vi "Tool Object.vi"(8 "error in (no error)":errorcluster, 11 "Tool Path in":refnum<class "Tool Path.lvclass">) -> (0 "error out":errorcluster, 2 "Points":T1[](array[typedef]), 3 "Tool Path out":refnum<class "Tool Path.lvclass">)   [LabVIEW 2019, in "Tool Path.lvclass"]
uses:
  Tool Path.lvclass
  Parse/PathCommands/Point.ctl
  Settings/ObjectSettings/ObjectSettings.lvclass/ObjectSettings.ctl
  Settings/Path Settings/Path Settings.lvclass
  C:/Users/Albro/Documents/GitHub/AFM-Lithography/lvsrc/Classes/Settings/ObjectSettings/ObjectSettings.lvclass
  Settings/ObjectSettings/ObjectSettings.lvclass
  Parse/PathCommands/PathCommands.lvclass
panel:
  out "Voltage Values":dbl[](array[numeric])
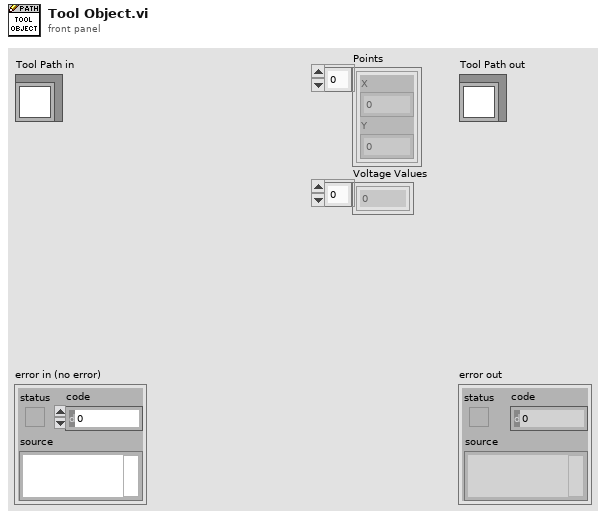
[diagram p1: front panel]
types:
  T1 = typedef "PathCommands.lvclass/Point.ctl" = cluster{"X":dbl, "Y":dbl}
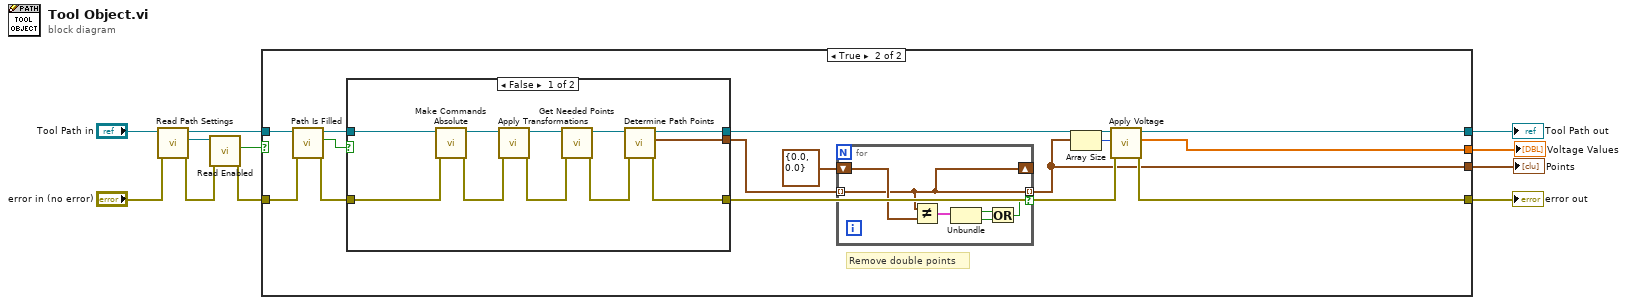
[diagram p0: block diagram]
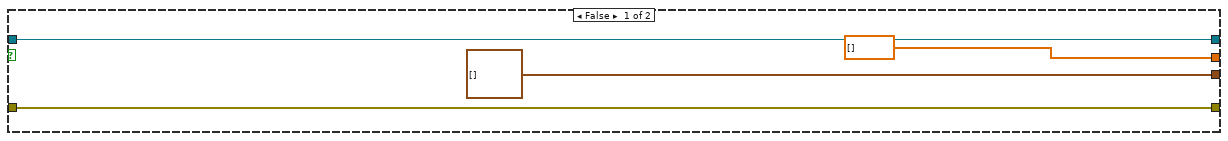
[diagram p2: hidden frame]
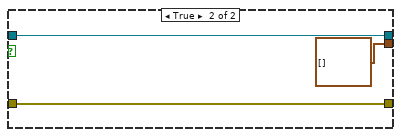
[diagram p3: hidden frame]
diagram:
  n1 = call-dynamic "Read Path Settings.vi"("error in (no error)"="error in (no error)", "Tool Path in"="Tool Path in") -> ("error out"=w4:errorcluster, "Path Settings.lvclass"=w10:refnum<class "Path Settings.lvclass">, "Tool Path out"=w9:refnum<class "Tool Path.lvclass">)  [unwired: 7 in]
  n2 = call "Read Enabled.vi"("error in (no error)"=w4, "ObjectSettings in"=w10) -> ("error out"=w3:errorcluster, "Enabled"=w6:bool)  [unwired: 7 in, 1 out]
  n3 = case shown="True" w6 {
    tunnel: w9 -> [w15 w28]
    tunnel: [w15 w23] -> w8
    tunnel: w3 -> [w14 w25]
    tunnel: [w14 w21] -> w7
    tunnel: [T1[] [] ("Points") w18] -> w2
    tunnel: [dbl[] [] ("Voltage Values") w16] -> w1
    frame False {
    }
    frame True {
      # "Remove double points"
      n4 = call "Path Is Filled.vi"("error in (no error)"=w25, "Tool Path in"=w28) -> ("error out"=w26:errorcluster, "Filled?"=w27:bool, "Tool Path out"=w29:refnum<class "Tool Path.lvclass">)  [unwired: 7 in]
      n5 = case shown="False" w27 {
        tunnel: w29 -> [w46 w49]
        tunnel: [w42 w49] -> w24
        tunnel: w26 -> [w41 w48]
        tunnel: [w37 w48] -> w22
        tunnel: [w36 T1[] [] ("Points")] -> w17
        frame False {
          n6 = call "Make Commands Absolute.vi"("error in (no error)"=w41, "Tool Path in"=w46) -> ("error out"=w40:errorcluster, "Tool Path out"=w43:refnum<class "Tool Path.lvclass">)  [unwired: 8 in]
          n7 = call-dynamic "Apply Transformations.vi"("error in (no error)"=w40, "Tool Path in"=w43) -> ("error out"=w39:errorcluster, "Tool Path out"=w45:refnum<class "Tool Path.lvclass">)  [unwired: 8 in]
          n8 = call-dynamic "Get Needed Points.vi"("error in (no error)"=w39, "Tool Path in"=w45) -> ("error out"=w38:errorcluster, "Tool Path out"=w44:refnum<class "Tool Path.lvclass">)  [unwired: 8 in]
          n9 = call-dynamic "Determine Path Points.vi"("error in (no error)"=w38, "Tool Path in"=w44) -> ("error out"=w37:errorcluster, "Points"=w36:T1[], "Tool Path out"=w42:refnum<class "Tool Path.lvclass">)  [unwired: 7 in]
        }
        frame True {
        }
      }
      n10 = for {
        tunnel: w17 -> [w34] mode=indexing
        tunnel: [w34] -> w18 mode=indexing if=w30
        shift-right: [w34] -> _
        shift-left: T1 {"X"=0.0, "Y"=0.0} ("Point") -> [w35]
        n11 = Not Equal?(x=w34, y=w35) -> (x != y?=w33:cluster{"X":bool, "Y":bool})
        n12 = Unbundle(w33) -> ("X"=w32:bool, "Y"=w31:bool)
        n13 = Or(x=w32, y=w31) -> (x .or. y?=w30:bool)
      }
      n14 = Array Size(array=w18) -> (size(s)=w20:i32)
      n15 = call-dynamic "Apply Voltage.vi"("error in (no error)"=w22, "Number of Points"=w20, "Tool Path in"=w24) -> ("error out"=w21:errorcluster, "Voltage Values"=w16:dbl[], "Tool Path out"=w23:refnum<class "Tool Path.lvclass">)  [unwired: 6 in]
    }
  }
  "error out" <- w7
  "Tool Path out" <- w8
  "Points" <- w2
  "Voltage Values" <- w1
